vi "MGCC_StaEst_initial_2.vi"() -> ()   [LabVIEW 2016]
uses:
  <vilib>/imath/engines/lvmath2/RunTimeEngine/RunTimeType/NIMS_RunTimeType_From StrictType (excl LVString).vi
  <instcachedir>/0/NIMS_RunTimeType_From StrictType (excl LVString)_BBF44FB49F834B71AF7A14CCEDF8BECD.lvgen/NIMS_RunTimeType_From StrictType (excl LVString)_BBF44FB49F834B71AF7A14CCEDF8BECD_024.vi
  <vilib>/imath/engines/lvmath2/RunTimeEngine/Struct/NIMS_StructSetField.vi
  <vilib>/imath/engines/lvmath2/RunTimeEngine/IndexRead/NIMS M($,R2).vi
  <instcachedir>/0/NIMS M($,R2)_D9380E19261A4ADFB2D364AF6959C6EF.lvgen/NIMS M($,R2)_D9380E19261A4ADFB2D364AF6959C6EF_001.vi
  <instcachedir>/0/NIMS_RunTimeType_From StrictType (excl LVString)_BBF44FB49F834B71AF7A14CCEDF8BECD.lvgen/NIMS_RunTimeType_From StrictType (excl LVString)_BBF44FB49F834B71AF7A14CCEDF8BECD_009.vi
  <vilib>/imathl/engines/lvmath/Functions/Error Handling/Create Error.vi
  <vilib>/imath/engines/lvmath2/RunTimeEngine/BuiltInFunctions/size/NIMS_I32=size(GCol,I32).vi
  <instcachedir>/0/NIMS_I32=size(GCol,I32)_3BEAC9C04C22472CB193ADA08E7FE41C.lvgen/NIMS_I32=size(GCol,I32)_3BEAC9C04C22472CB193ADA08E7FE41C_000.vi
  <vilib>/imath/engines/lvmath2/RunTimeEngine/RangeToken/NIMS_Range_R2 - Integer.vi
  <instcachedir>/0/NIMS_Range_R2 - Integer_89B873E74E6E489885E44F751DD9C6BF.lvgen/NIMS_Range_R2 - Integer_89B873E74E6E489885E44F751DD9C6BF_000.vi
  <vilib>/imath/engines/lvmath2/RunTimeEngine/CommandStatement/MC_CommandStatement_break.vi
  <vilib>/imath/engines/lvmath2/RunTimeEngine/IndexRead/NIMS V(S).vi
  <instcachedir>/0/NIMS V(S)_0488751826AF41519A22953C041130DC.lvgen/NIMS V(S)_0488751826AF41519A22953C041130DC_002.vi
  <vilib>/imath/engines/lvmath2/RunTimeEngine/MatrixToken/NIMS_MatrixToken_M_RV.vi
  <instcachedir>/0/NIMS_MatrixToken_M_RV_EE14907D4B194E829889005D2F556E9C.lvgen/NIMS_MatrixToken_M_RV_EE14907D4B194E829889005D2F556E9C_002.vi
  <vilib>/imath/engines/lvmath2/RunTimeEngine/ErrorHandling/NIMS_Create Error From Enums.vi
  <vilib>/imath/engines/lvmath2/RunTimeEngine/NodeEndStatement/NIMS_NodeEndStatement_Output.vi
  <instcachedir>/0/NIMS_NodeEndStatement_Output_53EC0D466D134D7ABD903AC30B43404B.lvgen/NIMS_NodeEndStatement_Output_53EC0D466D134D7ABD903AC30B43404B_013.vi
  <vilib>/imath/engines/lvmath2/RunTimeEngine/ErrorHandling/NIMS_Finalize Error.vi
panel:
  out "Loc1":cluster{"Zeroinj":i32[][]}
  out "Loc":cluster{"Zeroinj":i32[][], "Line":i32[][]}
  out "Num1":cluster{"Zeroinj":i32}
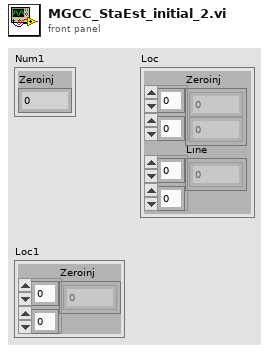
[diagram p1: front panel]
types:
  T1 = cluster{"VOL":cdb[][], "PN":dbl[][], "QN":dbl[][], "IN":dbl[][], "Ve":dbl[][], "Vf":dbl[][], "VN":dbl[][], "AN":dbl[][]}
  T2 = cluster{"topology":dbl[][], "Configurations":dbl[][], "Loads":dbl[][], "Slack":dbl, "Vpu_slack_phase":cdb[], "Vnom":dbl, "Graphic":dbl[][], "NumN":dbl, "NumL":dbl, "NumC":dbl, "NumZ":dbl, "NumR":dbl, "NumS":dbl, "Nodes_ID":dbl[], "BLIN":cdb[][][], "ZLIN":cdb[][][]}
  T3 = cluster{"Node":dbl, "Line":dbl, "StateVar":i32, "Zeroinj":i32}
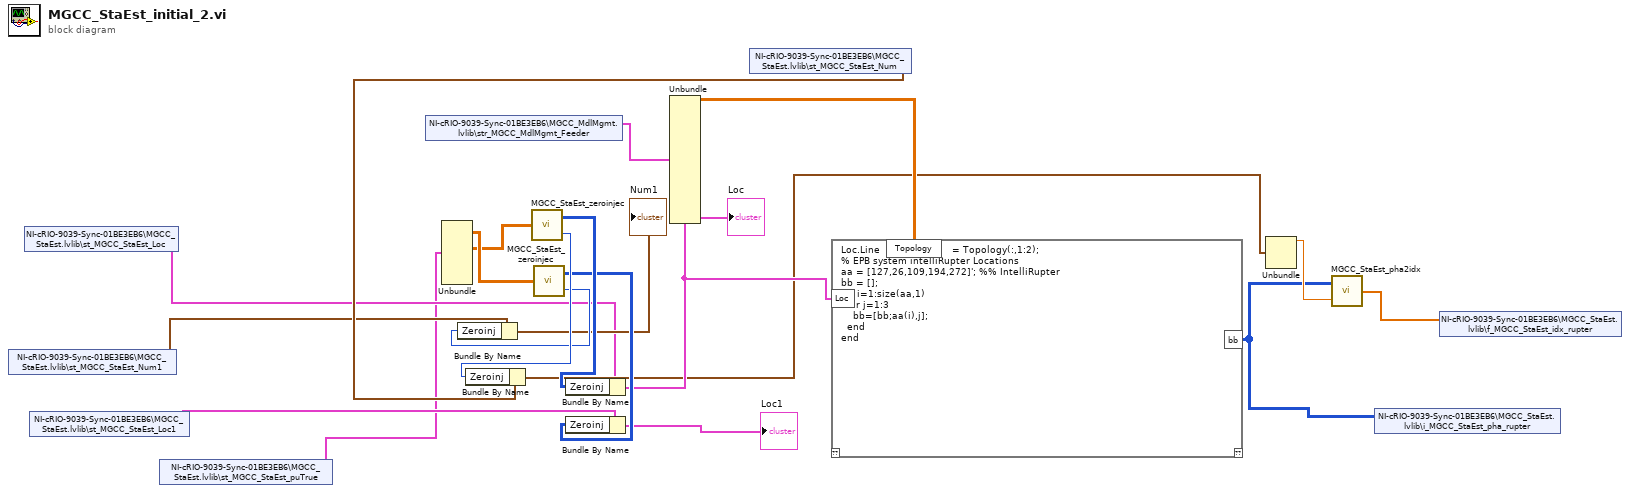
[diagram p0: block diagram]
diagram:
  n1 = shared-variable "NI-cRIO-9039-Sync-01BE3EB6\\MGCC_StaEst.lvlib\\st_MGCC_StaEst_Num1"() -> (w5:cluster{"Zeroinj":i32})  [unwired: 1 in, 1 out]
  n2 = shared-variable "NI-cRIO-9039-Sync-01BE3EB6\\MGCC_StaEst.lvlib\\st_MGCC_StaEst_Loc"() -> (w6:cluster{"Zeroinj":i32[][], "Line":i32[][]})  [unwired: 1 in, 1 out]
  n3 = shared-variable "NI-cRIO-9039-Sync-01BE3EB6\\MGCC_StaEst.lvlib\\st_MGCC_StaEst_Loc1"() -> (w4:cluster{"Zeroinj":i32[][]})  [unwired: 1 in, 1 out]
  n4 = shared-variable "NI-cRIO-9039-Sync-01BE3EB6\\MGCC_StaEst.lvlib\\st_MGCC_StaEst_puTrue"() -> (w3:T1)  [unwired: 1 in, 1 out]
  n5 = shared-variable "NI-cRIO-9039-Sync-01BE3EB6\\MGCC_MdlMgmt.lvlib\\str_MGCC_MdlMgmt_Feeder"() -> (w10:T2)  [unwired: 1 in, 1 out]
  n6 = Unbundle(w3) -> ("PN"=w20:dbl[][], "IN"=w19:dbl[][])  [unwired: 6 out]
  n7 = call "MGCC_StaEst_zeroinjec.vi"("A"=w19) -> ("Node_ZeroInjec"=w16:i32[][], "Num_ZeroInjec"=w18:i32)
  n8 = call "MGCC_StaEst_zeroinjec.vi"("A"=w20) -> ("Node_ZeroInjec"=w15:i32[][], "Num_ZeroInjec"=w17:i32)
  n9 = Bundle By Name(cluster=w5, "Zeroinj"=w17) -> (→"Num1":cluster{"Zeroinj":i32})
  n10 = Bundle By Name(cluster=w6, "Zeroinj"=w16) -> (w12:cluster{"Zeroinj":i32[][], "Line":i32[][]})
  "Loc" <- w12
  n11 = Bundle By Name(cluster=w4, "Zeroinj"=w15) -> (→"Loc1":cluster{"Zeroinj":i32[][]})
  n12 = Unbundle(w10) -> ("topology"=w9:dbl[][])  [unwired: 15 out]
  n13 = shared-variable "NI-cRIO-9039-Sync-01BE3EB6\\MGCC_StaEst.lvlib\\st_MGCC_StaEst_Num"() -> (w7:T3)  [unwired: 1 in, 1 out]
  n14 = Bundle By Name(cluster=w7, "Zeroinj"=w18) -> (w8:T3)
  n15 = mathscript code="Loc.Line                        = Topology(:,1:2);\n% EPB system intelliRupter Locations\naa = [127,26,109,194,272]'; %% IntelliRupter\nbb = [];\nfor i=1:size(aa,1)\n  for j=1:3\n    bb=[bb;aa(i),j];\n  end\nend"("Loc"=w12, "Topology"=w9) -> ("bb"=w1:i32[][])  [unwired: 1 in, 1 out]
  n16 = Unbundle(w8) -> ("Node"=w11:dbl)  [unwired: 3 out]
  n17 = call "MGCC_StaEst_pha2idx.vi"("n"=w11, "byphase"=w1) -> ("index"=w2:dbl[])
  n18 = shared-variable "NI-cRIO-9039-Sync-01BE3EB6\\MGCC_StaEst.lvlib\\i_MGCC_StaEst_pha_rupter"(w1) -> ()  [unwired: 1 in, 1 out]
  n19 = shared-variable "NI-cRIO-9039-Sync-01BE3EB6\\MGCC_StaEst.lvlib\\f_MGCC_StaEst_idx_rupter"(w2) -> ()  [unwired: 1 in, 1 out]
